vi "niDTS WLAN DSSS Rx Test Get Default Parameters.vi"(0 "Dummy Test Handle in":T6, 11 "error in (no error)":errorcluster) -> (4 "Dummy Test Handle out":T6, 8 "Default Parameters":T1={"DSSS Data Rate (Mbps)"=enum."1", "Chains"=[TRUE, FALSE, FALSE, FALSE], "Bandwidth (Hz)"=enum."20 MHz", "Channel"=1, "Power (dBm)"=1.0, "16 symbols"=TRUE, "Payload Length (bytes)"=0, "Idle Interval (s)"=1.0, "External Attenuation (dB)"=[0.0, 0.0, 0.0, 0.0], "RX Measurement Parameters"={"Number of Packets"=1000, "MacAddress"="FF:FF:FF:FF:FF:FF"}} {"Idle Interval (s)" format="%_3p"; "Channel" items=["1"=1, "2"=2, "3"=3, "4"=4, "5"=5, "6"=6, "7"=7, "8"=8, "9"=9, "10"=10, "11"=11, "12"=12, "13"=13, "14"=14]}, 15 "error out":errorcluster)   [LabVIEW 2014, in "niDTS WLAN.lvlib"]
uses:
  niDTS WLAN.lvlib
  Rx Test/Includes/niDTS WLAN Rx Test INC Handle.ctl
  Rx Test/Objects/BASE_class/niDTS WLAN Rx Test.lvclass
  Includes/niDTS WLAN Rx Test INC DSSS Parameters.ctl
  Includes/niDTS WLAN INC DSSS Data Rate.ctl
  Includes/niDTS WLAN INC CH BW DSSS.ctl
  Includes/niDTS WLAN INC Channel DSSS.ctl
  Rx Test/Includes/niDTS WLAN INC RX Measurement Parameters.ctl
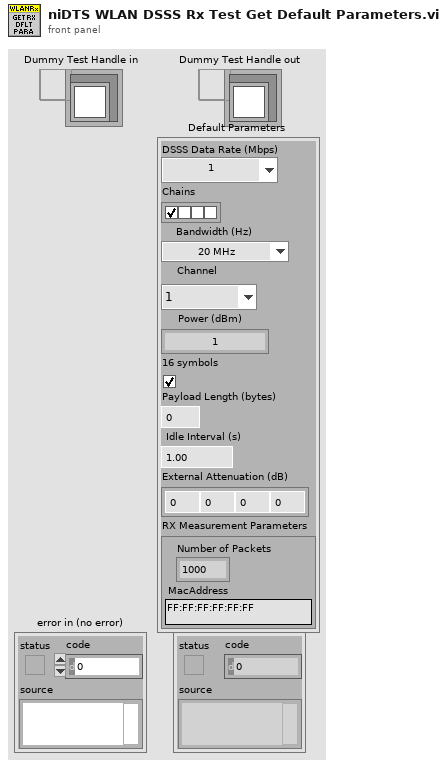
[diagram p1: front panel]
types:
  T1 = typedef "niDTS WLAN.lvlib/niDTS WLAN Rx Test INC DSSS Parameters.ctl" = cluster{"DSSS Data Rate (Mbps)":T2, "Chains":bool[], "Bandwidth (Hz)":T3, "Channel":T4, "Power (dBm)":dbl, "16 symbols":bool, "Payload Length (bytes)":i32, "Idle Interval (s)":dbl, "External Attenuation (dB)":dbl[], "RX Measurement Parameters":T5}
  T2 = typedef "niDTS WLAN.lvlib/niDTS WLAN INC DSSS Data Rate.ctl" = enum16{"1", "2", "5.5", "11"}
  T3 = typedef "niDTS WLAN.lvlib/niDTS WLAN INC CH BW DSSS.ctl" = enum16{"20 MHz"}
  T4 = typedef "niDTS WLAN.lvlib/niDTS WLAN INC Channel DSSS.ctl" = i8
  T5 = typedef "niDTS WLAN.lvlib/niDTS WLAN INC RX Measurement Parameters.ctl" = cluster{"Number of Packets":i32, "MacAddress":string}
  T6 = typedef "niDTS WLAN.lvlib/niDTS WLAN Rx Test INC Handle.ctl" = refnum<data-value>
  T7 = typedef "niDTS WLAN.lvlib/niDTS WLAN Rx Test INC Parameters.ctl" = cluster{"Standard":T8, "DSSS Data Rate (Mbps)":T2, "OFDM Data Rate (Mbps)":T9, "MCS Index":i32, "N Spatial Streams":i32, "Chains":bool[], "Bandwidth (Hz)":T10, "Channel":i32, "Power (dBm)":dbl, "Guard Interval":T11, "FEC Coding":T12, "16 symbols":bool, "Payload Length (bytes)":i32, "Idle Interval (s)":dbl, "External Attenuation (dB)":dbl[], "RX Measurement Parameters":T5}
  T8 = typedef "niDTS WLAN.lvlib/niDTS WLAN INC Standard.ctl" = enum16{"802.11 b DSSS", "802.11 a/g OFDM", "802.11 n HT", "802.11 ac VHT"}
  T9 = typedef "niDTS WLAN.lvlib/niDTS WLAN INC OFDM Data Rate.ctl" = enum16{"6", "9", "12", "18", "24", "36", "48", "54"}
  T10 = typedef "niDTS WLAN.lvlib/niDTS WLAN INC CH BW.ctl" = enum16{"20 MHz", "40 MHz", "80 MHz", "160 MHz"}
  T11 = typedef "niDTS WLAN.lvlib/niDTS WLAN INC GI.ctl" = enum16{"LONG", "SHORT"}
  T12 = typedef "niDTS WLAN.lvlib/niDTS WLAN INC FEC Coding.ctl" = enum16{"BCC", "LDPC"}
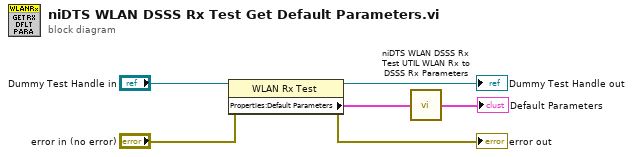
[diagram p0: block diagram]
diagram:
  n1 = property class="WLAN Rx Test"(reference="Dummy Test Handle in", error in="error in (no error)") -> (reference out=→"Dummy Test Handle out":T6, error out=→"error out":errorcluster, "Properties:Default Parameters"=w2:T7)
  n2 = call "niDTS WLAN DSSS Rx Test UTIL WLAN Rx to DSSS Rx Parameters.vi"("WLAN Tx Parameters"=w2) -> ("WLAN Rx OFDM Input Parameters"=→"Default Parameters":T1)  [unwired: 14 in]
